vi "LVClass_Pupil Resize Data.vi"(0 "Pupil in":refnum<class "Pupil.lvclass">, 5 "Factor":u8, 7 "Resized Pupil in":refnum<class "Pupil.lvclass">, 11 "error in (no error)":errorcluster) -> (4 "Pupil out":refnum<class "Pupil.lvclass">, 8 "Resized Pupil in 2":refnum<class "Pupil.lvclass">, 15 "error out":errorcluster)   [LabVIEW 2020, in "Pupil.lvclass"]
doc: "Set Pupil buffer.\n\n--------------------------------------------------------------------------------\n\n<B>PupilIn </B> : Pupil object.\n<B>PupilOut </B> : Pupil object.\n<B>data </B> : Pupil buffer to set.\n<B>ErrorIn </B> : Error\n<B>ErrorOut </B> : Error\n\n--------------------------------------------------------------------------------"
uses:
  Pupil.lvclass
  Pupil.lvclass/Pupil.ctl
  LVClass_Pupil Read Pupil.vi
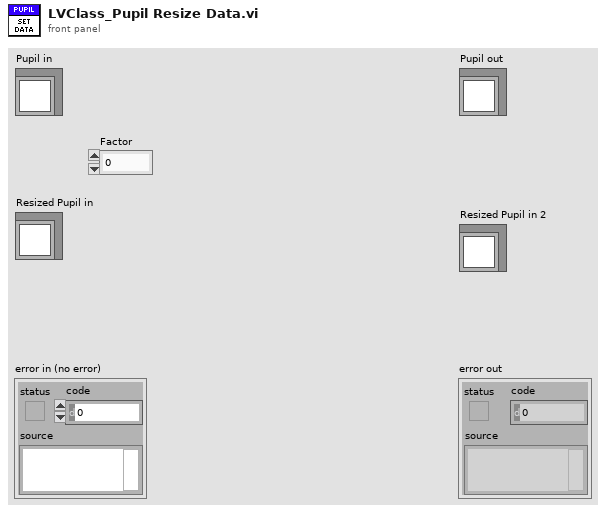
[diagram p1: front panel]
types:
  T1 = typedef "ClassID.ctl" = i64
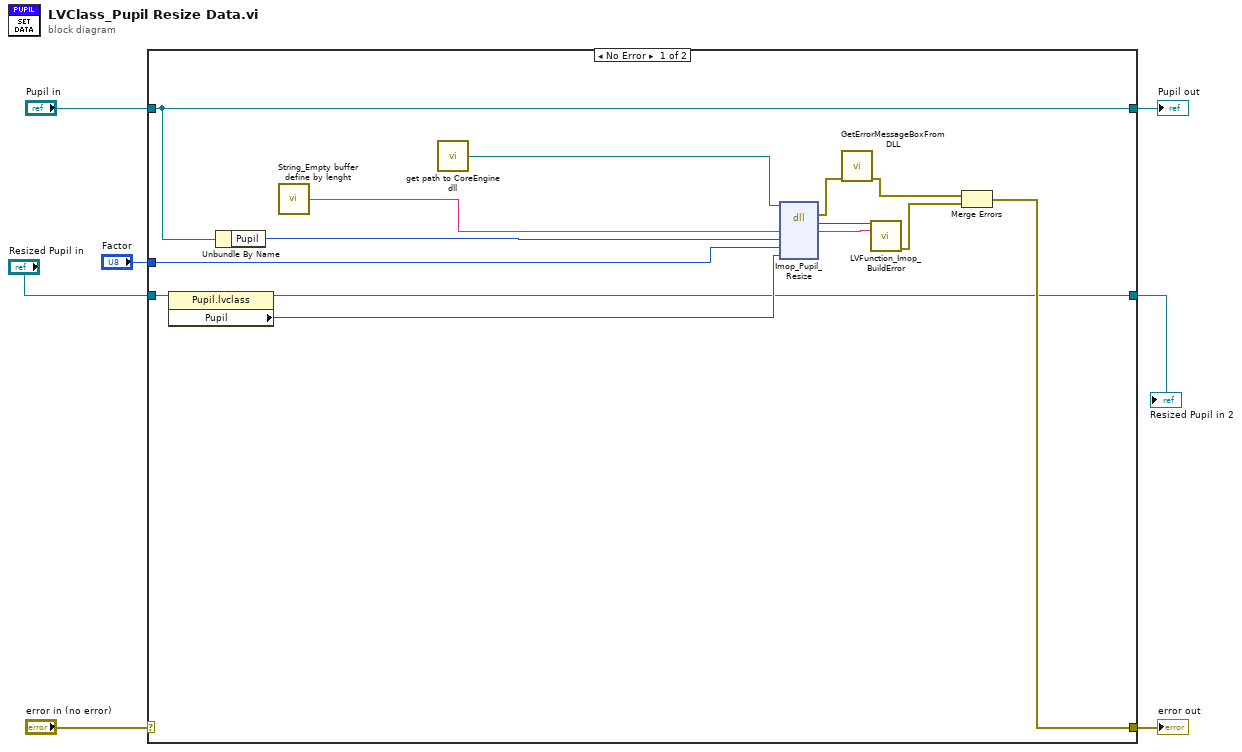
[diagram p0: block diagram]
diagram:
  n1 = case shown="No Error" "error in (no error)" {
    selector: "error in (no error)" -> [_ w24]
    tunnel: [w12 w24] -> w7
    tunnel: [w16 w23] -> w6
    tunnel: "Pupil in" -> [w16 w23]
    tunnel: "Resized Pupil in" -> [w11 w22]
    tunnel: [w9 w22] -> w4
    tunnel: "Factor" -> [w8 _]
    frame No Error {
      n2 = property class="Pupil.lvclass"(reference=w11) -> (reference out=w9:refnum<class "Pupil.lvclass">, "Pupil"=w10:T1)  [unwired: 1 in, 1 out]
      n3 = Unbundle By Name(w16) -> ("Pupil"=w15:T1)
      n4 = call "String_Empty buffer define by lenght.vi"() -> ("Empty buffer"=w21:string)  [unwired: 1 in]
      n5 = call "get path to CoreEngine dll.vi"() -> ("path to wavekit library"=w18:path)  [unwired: 14 in, 1 out]
      n6 = dll-call lib="D:/2_trunk/Soft_haso/ImOpCoreEngine4_LV2011/DLLs/ImopEngine4_vc100.dll" fn="Imop_Pupil_Resize"(path in=w18, "message"=w21, "pupil"=w15, "factor"=w8, "resized pupil"=w10) -> (error out=w17:errorcluster, "return type"=w19:i32, "message"=w20:string)  [unwired: 5 in, 1 out]
      n7 = call "GetErrorMessageBoxFromDLL.vi"("error IN"=w17) -> ("error OUT"=w14:errorcluster)  [unwired: 10 in]
      n8 = call "LVFunction_Imop_BuildError.vi"("code"=w19, "String to Prepend to source (\"\")"=w20) -> ("error out"=w13:errorcluster)  [unwired: 13 in]
      n9 = Merge Errors(w14, w13) -> (w12:errorcluster)
    }
    frame Error {
    }
  }
  "error out" <- w7
  "Pupil out" <- w6
  "Resized Pupil in 2" <- w4
